vi "FIB realtime imaging PXIe-6124.vi"(0 "HW Config":T4={"FIB X coil"="FIB/ao0", "FIB Y coil"="FIB/ao1", "Beam blank"="FIB/port0/line0", "Ext Scan"="FIB/port0/line1", "Detector"="FIB/ai1", "Post #1up"="PXI1Slot2/ao0", "Post #1down"="PXI1Slot2/ao1", "Post #2up"="PXI1Slot2/ao2", "Post #2down"="PXI1Slot2/ao3"}, 1 "Options":T3 {"Scan mode" items=["Raster", "Serpentine"]; "Det" items=["Detector A", "Detector B"]}, 2 "Single scan":bool, 3 "Scan Para":T2={"X resolution"=512, "Z resolution"=512, "X center"=0.0, "Z center"=0.0, "X size (V)"=10.0, "Z size (V)"=10.0, "Frame line rampdown ratio"=-0.1, "Scan rate (Hz)"=2000000, "Oversampling"=2} {"Frame line rampdown ratio" min=-1.0 max=1.0 step=0.05 format="%.2g"; "Scan rate (Hz)" max=4000000 format="%#.6p"}, 4 "As subVi":bool, 5 "COM port":refnum<visa-resource-name>="COM1") -> (7 "Info & Status":T1={"Actual scan rate"=2000000.0, "X resolution with rampdown"=552, "Actual sample rate"=4000000.0, "Fetch backlog"=664878.0, "Total scan points"=276000, "Frame rate (/s)"=7} {"Fetch backlog" format="%#_6p"; "Actual sample rate" format="%#_6p"; "Actual scan rate" format="%#_4p"}, 10 "error out":errorcluster)   [LabVIEW 2018]
uses:
  <vilib>/DAQmx/write.llb/DAQmx Write (Analog 1D DBL NChan 1Samp).vi
  <vilib>/DAQmx/write.llb/DAQmx Write (Digital Wfm 1Chan NSamp).vi
  <vilib>/DAQmx/write.llb/DAQmx Write (Analog 2D DBL NChan NSamp).vi
  <vilib>/DAQmx/read.llb/DAQmx Read (Raw 1D I16).vi
  <vilib>/Analysis/2dsp.llb/Decimate (single shot, DBL).vi
  <vilib>/DAQmx/create/channels.llb/DAQmx Create Channel (AI-Voltage-Basic).vi
  <vilib>/DAQmx/create/channels.llb/DAQmx Create Channel (AO-Voltage-Basic).vi
  <vilib>/DAQmx/miscellaneous.llb/DAQmx Fill In Error Info.vi
  <vilib>/Waveform/DWDTOps.llb/DWDT Invert Digital.vi
  <vilib>/DAQmx/configure/timing.llb/DAQmx Timing (Sample Clock).vi
  <vilib>/DAQmx/create/channels.llb/DAQmx Create Channel (DO-Digital Output).vi
  <vilib>/DAQmx/create/channels.llb/DAQmx Create Channel (CO-Pulse Generation-Frequency).vi
  <vilib>/DAQmx/configure/trigger.llb/DAQmx Start Trigger (Digital Edge).vi
  <vilib>/Waveform/DWDTOps.llb/DWDT Uncompress Digital.vi
  <vilib>/Waveform/DWDTOps.llb/Digital Pattern Generator (Single Value).vi
  <vilib>/Analysis/NI_AALPro.lvlib
  <resource>/objmgr/daqmx.rc
panel:
  in  "Spot":bool
  in  "Api":refnum<k7>(container)
  out "Image shift":u32
  out "AI SampleClk.MaxRate":dbl
  in  "Sweep enabled":bool
  in  "Focus (V)":dbl min=-10.0 max=10.0 step=0.1 format="%.3g"
  in  "Sweep rate (Hz)":dbl=0.5 min=0.01 step=0.1 format="%0.2f"
  in  "Level #":u8
  in  "Sweep direction":bool
  in  "Angle (V)":dbl min=-10.0 max=10.0 step=0.1 format="%.3g"
  in  "Position (V)":dbl min=-10.0 max=10.0 step=0.1 format="%.3g"
  in  "Imbalance (V)":dbl min=-10.0 max=10.0 step=0.1 format="%.3f"
  out "Post #2down":tag
  out "Post #2up":tag
  out "Post #1down":tag
  out "Post #1up":tag
  out "Low blanked":bool
  in  "Machine Type":u8(ring) items=["Feiss", "NVision", "Jeiss"]
  out "Ext scan":tag
  out "Detector":tag="PXI1Slot7/ai0"
  out "FIB Y coil":tag="PXI1Slot7/ao1"
  out "FIB X coil":tag="PXI1Slot7/ao0"
  in  "Beam blanked":bool
  out "Beam blank":tag="PXI1Slot7/port0/line0"
  out "Oversampling":u16=2
  out "Scan rate (Hz)":u32=2000000
  out "Frame line rampdown ratio":dbl=0.1
  out "Y end":dbl=1.0
  out "X end":dbl=1.0
  out "Y start":dbl=-1.0
  out "X start":dbl=-1.0
  out "Y resolution":u32=500
  out "X resolution":u32=500
  out "Flip z":bool
  out "Flip x":bool
  out "Scan mode":u16
  out "Live image":i16[][](graph)
  in  "stop":bool=TRUE
  # "Flip"
  # "Scan coils"
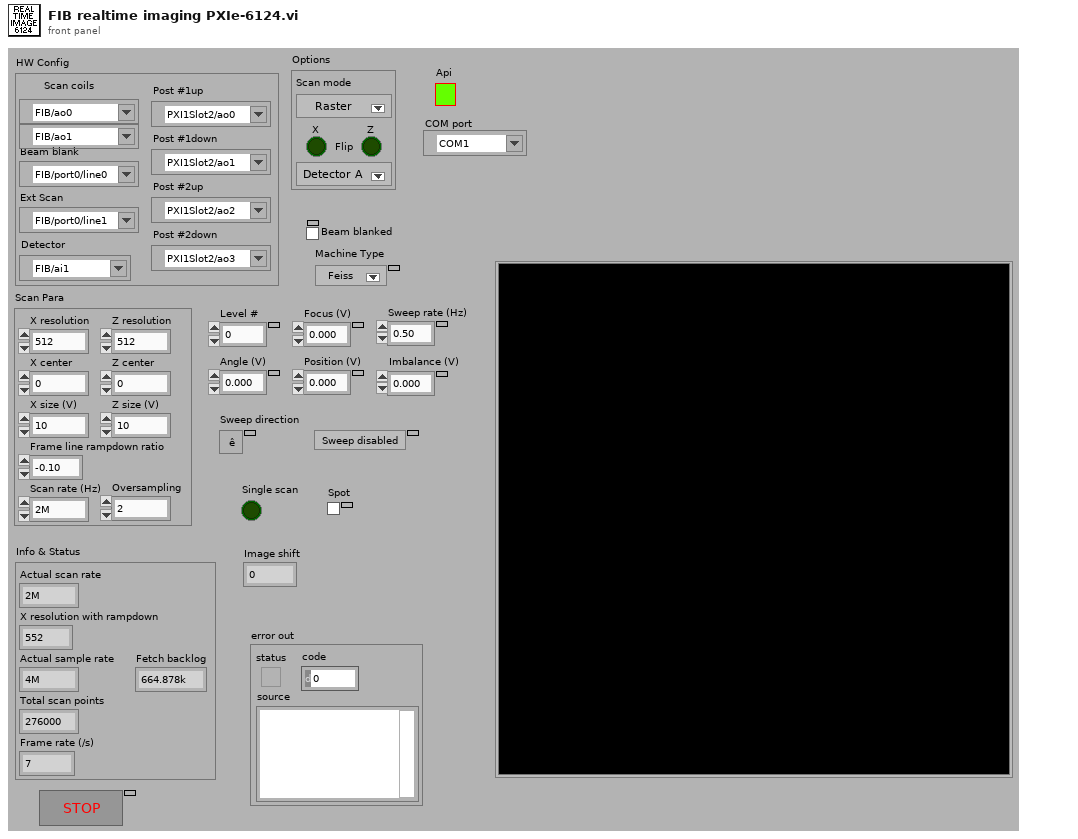
[diagram p1: front panel]
types:
  T1 = cluster{"Actual scan rate":dbl, "X resolution with rampdown":i32, "Actual sample rate":dbl, "Fetch backlog":dbl, "Total scan points":i32, "Frame rate (/s)":u32}
  T2 = cluster{"X resolution":u32, "Z resolution":u32, "X center":dbl, "Z center":dbl, "X size (V)":dbl, "Z size (V)":dbl, "Frame line rampdown ratio":dbl, "Scan rate (Hz)":u32, "Oversampling":u16}
  T3 = cluster{"Scan mode":u16, "Flip x":bool, "Flip z":bool, "Det":u16}
  T4 = cluster{"FIB X coil":tag, "FIB Y coil":tag, "Beam blank":tag, "Ext Scan":tag, "Detector":tag, "Post #1up":tag, "Post #1down":tag, "Post #2up":tag, "Post #2down":tag}
  T5 = enum16{"SEM", "FIB", "Milling", "SEM + FIB", "Mill + SEM", "SEM Drift Correction", "FIB Drift Correction", "No Beam", "External", "External + SEM"}
  T6 = enum16{"SEM", "FIB", "Mill", "SEM + FIB", "Mill + SEM", "Drift SEM", "Drift FIB", "None", "Ext", "Ext + SEM"}
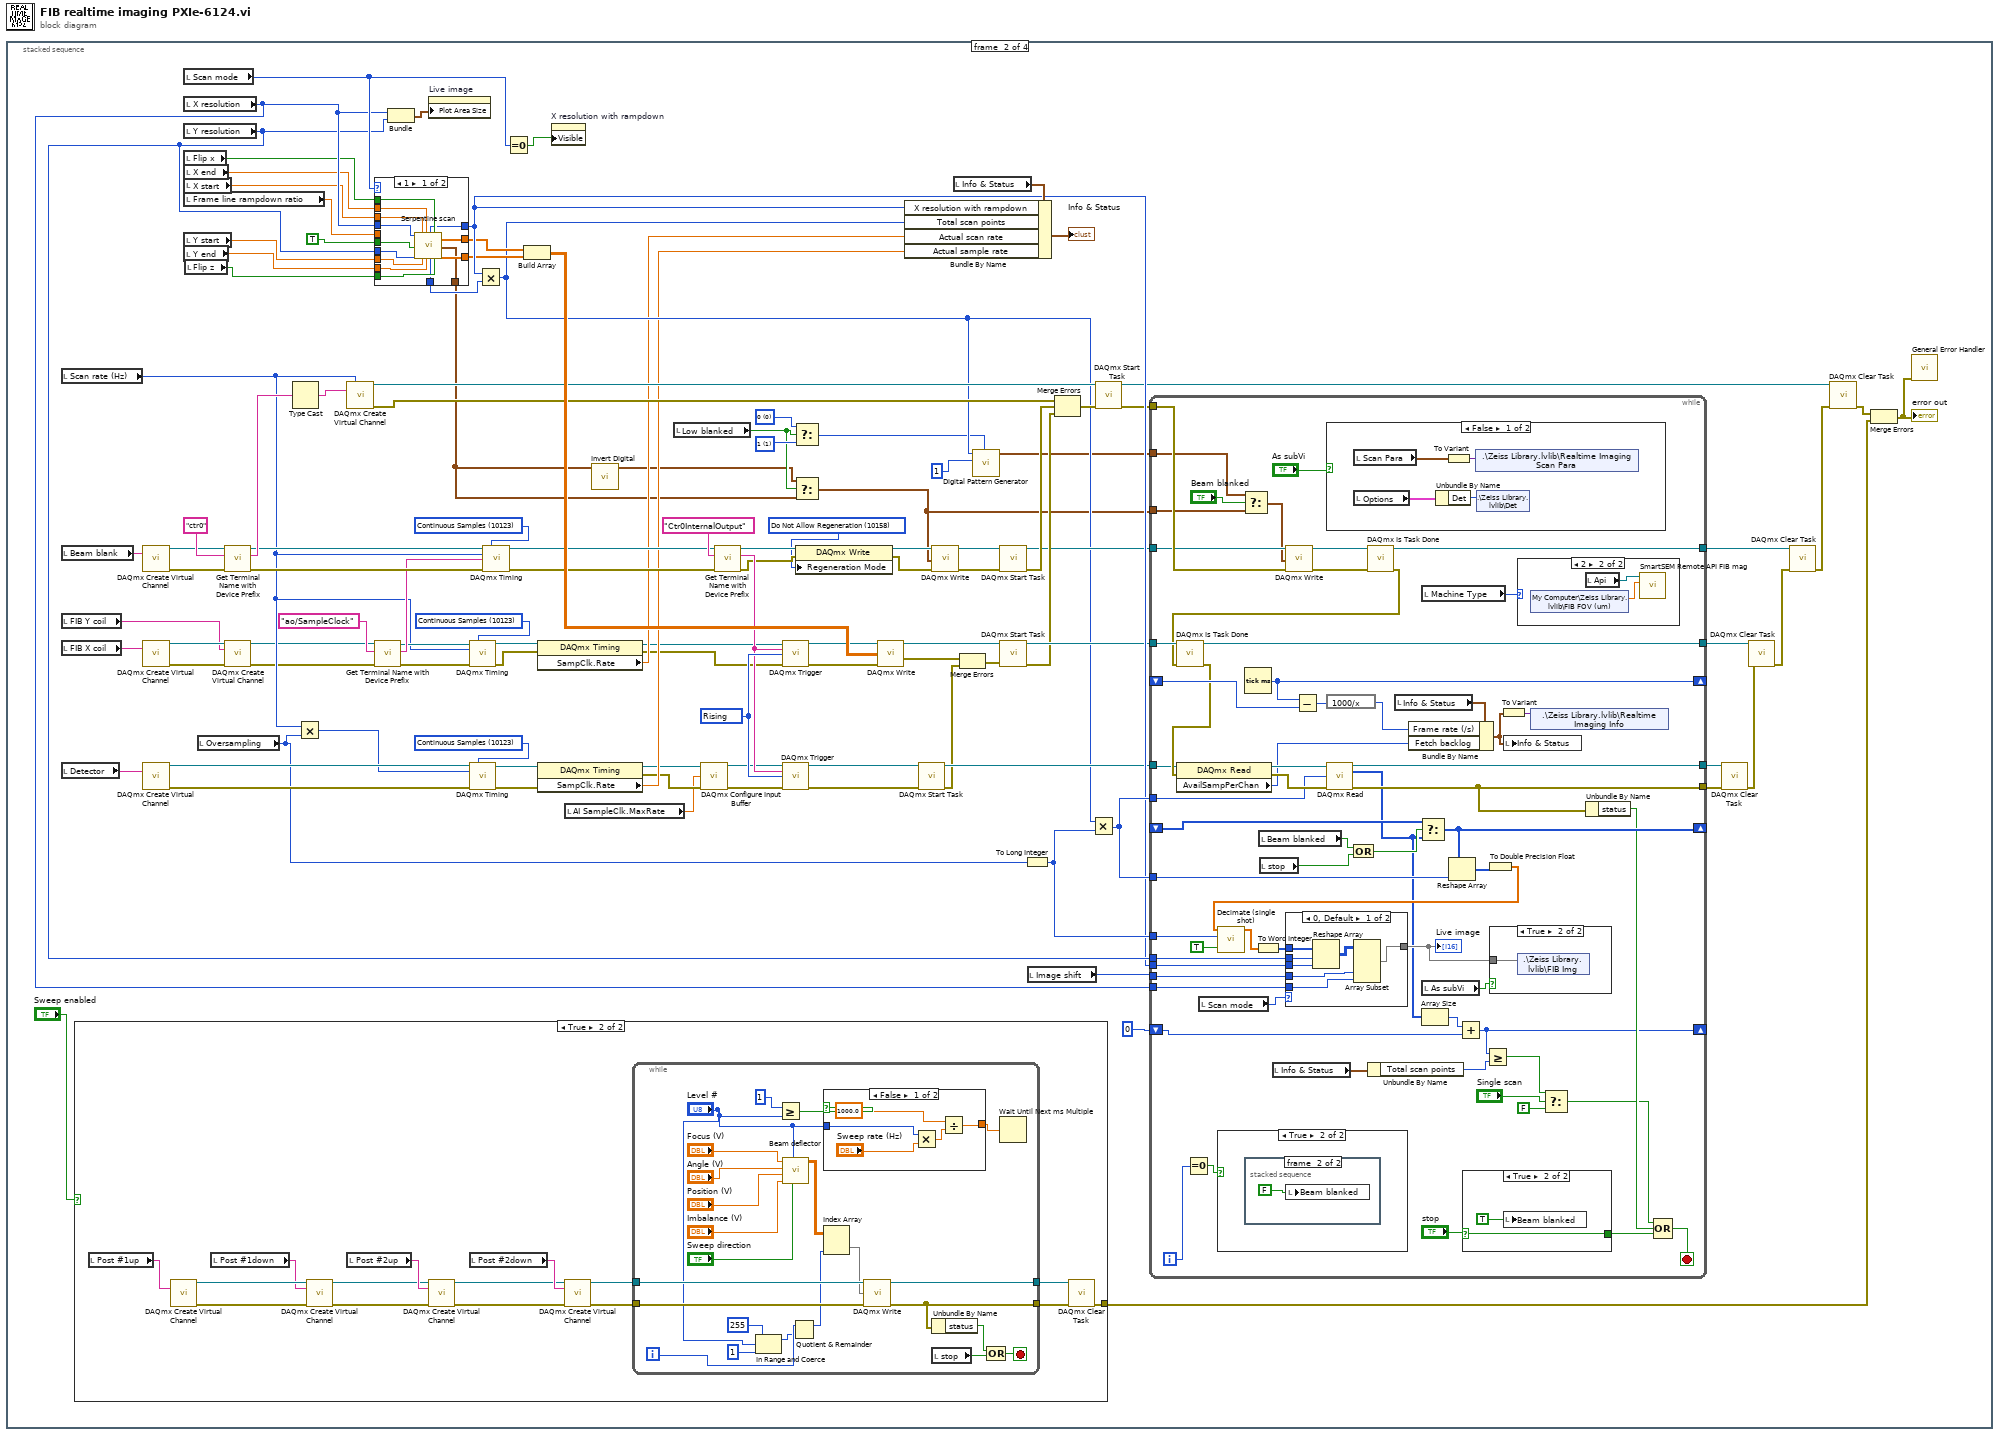
[diagram p0: block diagram]
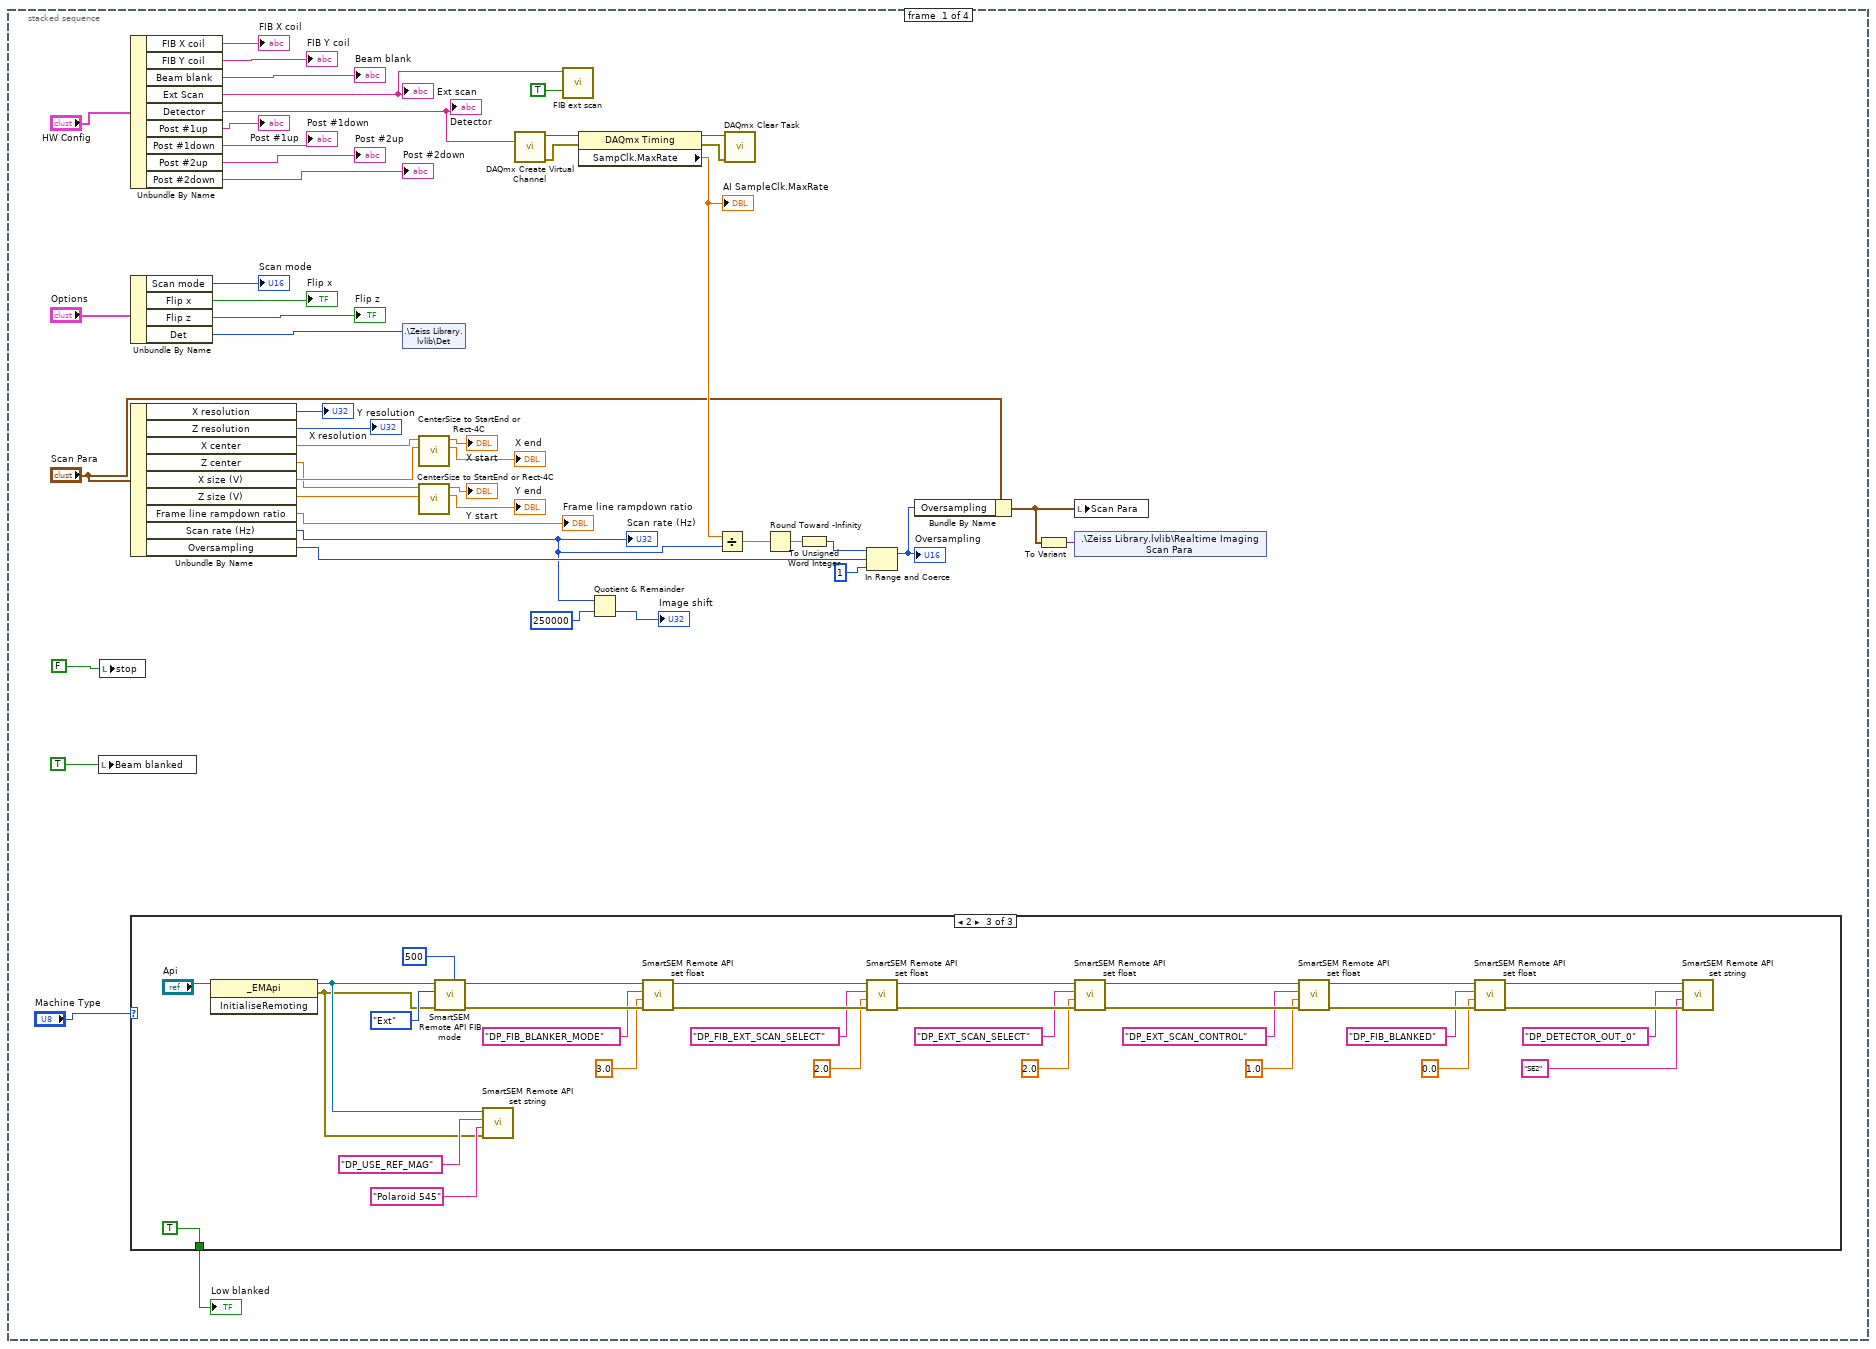
[diagram p2: hidden frame]
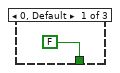
[diagram p3: hidden frame]
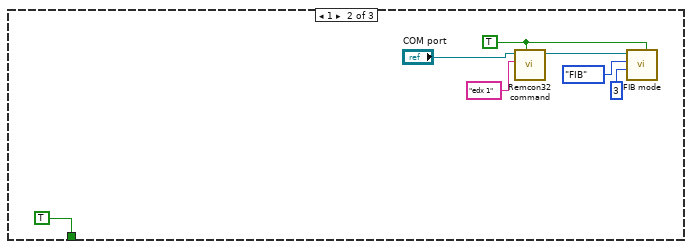
[diagram p4: hidden frame]
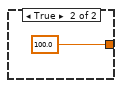
[diagram p6: hidden frame]
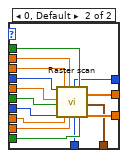
[diagram p7: hidden frame]
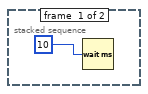
[diagram p11: hidden frame]
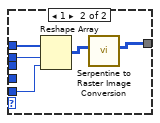
[diagram p14: hidden frame]
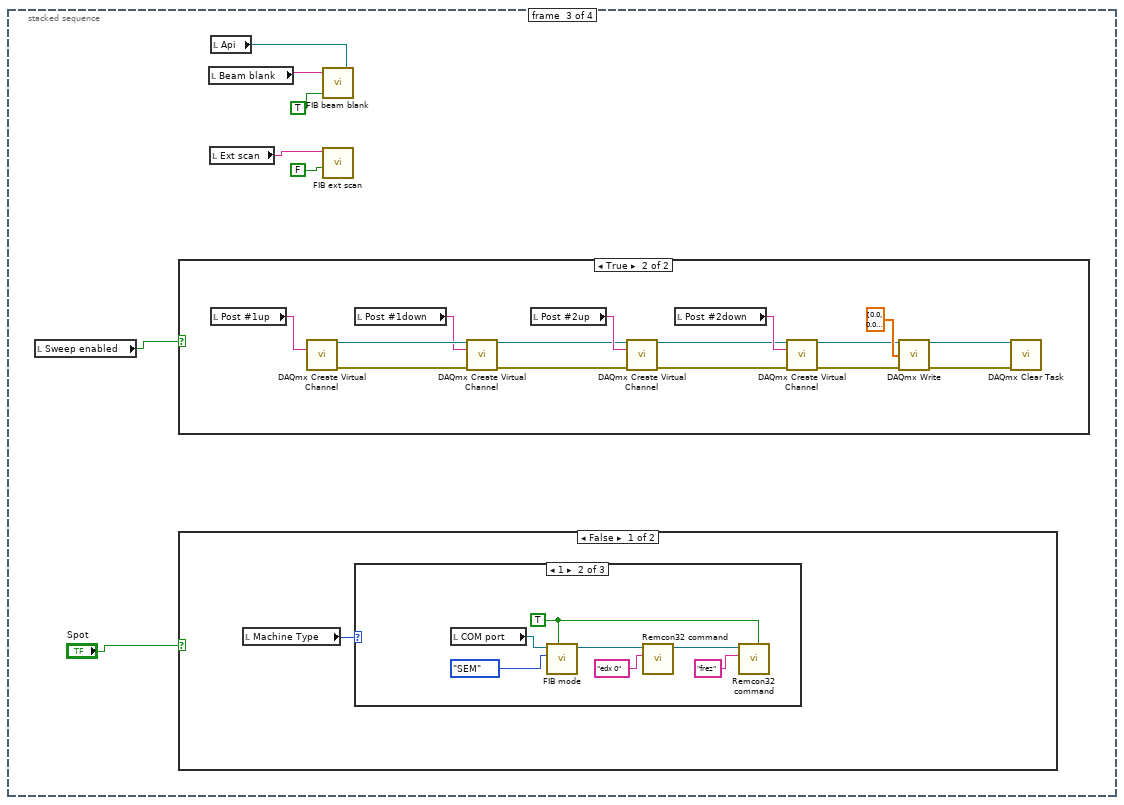
[diagram p15: hidden frame]
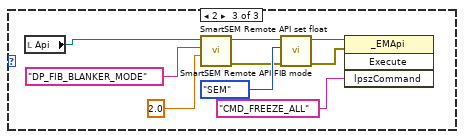
[diagram p17: hidden frame]
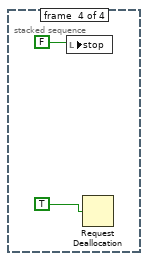
[diagram p20: hidden frame]
diagram:
  n1 = stacked-sequence {
    frame #0 {
      n2 = local write "Beam blanked"(TRUE ("Beam blanked")) -> ()
      n3 = local write "stop"(FALSE ("stop")) -> ()
      n4 = Unbundle By Name("HW Config") -> ("FIB X coil"=→"FIB X coil":tag, "FIB Y coil"=→"FIB Y coil":tag, "Beam blank"=→"Beam blank":tag, "Ext Scan"=w26:tag, "Detector"=w15:tag, "Post #1up"=→"Post #1up":tag, "Post #1down"=→"Post #1down":tag, "Post #2up"=→"Post #2up":tag, "Post #2down"=→"Post #2down":tag)
      "Detector" <- w15
      "Ext scan" <- w26
      n5 = Unbundle By Name("Options") -> ("Scan mode"=→"Scan mode":u16, "Flip x"=→"Flip x":bool, "Flip z"=→"Flip z":bool, "Det"=w40:u16)
      n6 = Unbundle By Name("Scan Para") -> ("X resolution"=→"X resolution":u32, "Z resolution"=→"Y resolution":u32, "X center"=w37:dbl, "Z center"=w33:dbl, "X size (V)"=w36:dbl, "Z size (V)"=w32:dbl, "Frame line rampdown ratio"=→"Frame line rampdown ratio":dbl, "Scan rate (Hz)"=w4:u32, "Oversampling"=w14:u16)
      "Scan rate (Hz)" <- w4
      n7 = case shown="2" "Machine Type" {
        tunnel: [FALSE ("Beam blanked") TRUE ("Beam blanked") TRUE ("Beam blanked")] -> w24
        frame 0, Default {
        }
        frame 1 {
          w53 = TRUE ("Close session")
          n8 = call "Remcon32 command.vi"("Initialization"=w53, "SEM command"="edx 1", "COM port in"="COM port") -> ("COM port out"=w52:refnum<visa-resource-name>)  [unwired: 5 in, 3 out]
          n9 = call "FIB mode.vi"("Close session"=w53, "Iterations"=u32 3, "FIB mode"=T5."FIB", "COM port in"=w52) -> ()  [unwired: 6 in, 2 out]
        }
        frame 2 {
          n10 = invoke class="_EMApi" method="InitialiseRemoting"(reference="Api") -> (reference out=w63:refnum<k7>, error out=w62:errorcluster)  [unwired: 2 in, 1 out]
          n11 = call "SmartSEM Remote API FIB mode.vi"("Wait (ms)"=u32 500, "error in"=w62, "FIB mode"=T6."Ext", "Api"=w63) -> ("error out"=w82:errorcluster, "Api out"=w83:refnum<k7>)  [unwired: 6 in]
          n12 = call "SmartSEM Remote API set string.vi"("error in"=w62, "vValue"="Polaroid 545" ("lpszParam"), "lpszParam"="DP_USE_REF_MAG", "Api"=w63) -> ()  [unwired: 6 in, 2 out]
          n13 = call "SmartSEM Remote API set float.vi"("error in"=w82, "vValue"=sgl 3.0, "lpszParam"="DP_FIB_BLANKER_MODE", "Api"=w83) -> ("error out"=w78:errorcluster, "Api out"=w79:refnum<k7>)  [unwired: 6 in]
          n14 = call "SmartSEM Remote API set float.vi"("error in"=w78, "vValue"=sgl 2.0, "lpszParam"="DP_FIB_EXT_SCAN_SELECT" ("lpszCommand"), "Api"=w79) -> ("error out"=w74:errorcluster, "Api out"=w75:refnum<k7>)  [unwired: 6 in]
          n15 = call "SmartSEM Remote API set float.vi"("vValue"=sgl 2.0, "lpszParam"="DP_EXT_SCAN_SELECT" ("lpszCommand")) -> ()  [unwired: 8 in, 2 out]
          n16 = call "SmartSEM Remote API set float.vi"("error in"=w74, "vValue"=sgl 1.0, "lpszParam"="DP_EXT_SCAN_CONTROL" ("lpszCommand"), "Api"=w75) -> ("error out"=w70:errorcluster, "Api out"=w71:refnum<k7>)  [unwired: 6 in]
          n17 = call "SmartSEM Remote API set float.vi"("error in"=w70, "vValue"=sgl 0.0, "lpszParam"="DP_FIB_BLANKED", "Api"=w71) -> ("error out"=w66:errorcluster, "Api out"=w67:refnum<k7>)  [unwired: 6 in]
          n18 = call "SmartSEM Remote API set string.vi"("error in"=w66, "vValue"="SE2" ("Det A Type"), "lpszParam"="DP_DETECTOR_OUT_0", "Api"=w67) -> ()  [unwired: 6 in, 2 out]
        }
      }
      "Low blanked" <- w24
      n19 = shared-variable ".\\Zeiss Library.lvlib\\Det"(w40) -> ()  [unwired: 1 in, 1 out]
      n20 = call "CenterSize to StartEnd or Rect-4C.vi"("Size"=w36, "Center"=w37) -> ("End"=→"X end":dbl, "Start"=→"X start":dbl)  [unwired: 3 in, 1 out]
      n21 = call "CenterSize to StartEnd or Rect-4C.vi"("Size"=w32, "Center"=w33) -> ("End"=→"Y end":dbl, "Start"=→"Y start":dbl)  [unwired: 3 in, 1 out]
      n22 = call-poly <vilib>:"DAQmx Create Virtual Channel.vi"("physical channels"=w15) -> ("task out"=w17:refnum<k21>, "error out"=w19:errorcluster)  [unwired: 8 in, 5 out]
      n23 = call "FIB ext scan.vi"("Ext on"=TRUE ("data"), "FIB Ext Scan"=w26) -> ()  [unwired: 9 in, 1 out]
      n24 = property class="DAQmx Timing"(reference=w17, error in=w19) -> (reference out=w16:refnum<k21>, error out=w18:errorcluster, "SampClk.MaxRate"=w12:dbl)
      "AI SampleClk.MaxRate" <- w12
      n25 = Quotient & Remainder(x=w4, y=u32 250000) -> (floor(x/y)=→"Image shift":u32)  [unwired: 1 out]
      n26 = Divide(x=w12, y=w4) -> (x/y=w11:dbl)
      n27 = call <vilib>:"DAQmx Clear Task.vi"("task in"=w16, "error in"=w18) -> ()  [unwired: 14 out]
      n28 = Round Toward -Infinity(1:w11) -> (0:w10:dbl)
      n29 = To Unsigned Word Integer(number=w10) -> (unsigned 16bit integer=w9:u16)
      n30 = In Range and Coerce(upper limit=w9, x=w14, lower limit=u16 1) -> (coerced(x)=w7:u16)  [unwired: 1 out]
      "Oversampling" <- w7
      n31 = Bundle By Name(cluster="Scan Para", "Oversampling"=w7) -> (w6:T2)
      n32 = To Variant(anything=w6) -> (Variant=w39:variant)
      n33 = local write "Scan Para"(w6) -> ()
      n34 = shared-variable ".\\Zeiss Library.lvlib\\Realtime Imaging Scan Para"(w39) -> ()  [unwired: 1 in, 1 out]
    }
    frame #1 {
      w105 = u8 1 items=["0", "1", "Z", "L", "H", "X", "T", "V"] ("value")
      w106 = u8 0 items=["0", "1", "Z", "L", "H", "X", "T", "V"] ("value")
      w117 = 10158 items=["Allow Regeneration"=10097, "Do Not Allow Regeneration"=10158] ("RegenMode")
      w142 = 10123 items=["Finite Samples"=10178, "Continuous Samples"=10123] ("sample mode")
      w130 = 10280 items=["Rising"=10280, "Falling"=10171] ("edge")
      w173 = 10123 items=["Finite Samples"=10178, "Continuous Samples"=10123, "Hardware Timed Single Point"=12522] ("sample mode")
      w177 = 10123 items=["Finite Samples"=10178, "Continuous Samples"=10123, "Hardware Timed Single Point"=12522] ("sample mode")
      n35 = local read "Scan rate (Hz)"() -> (w123:u32)
      n36 = local read "Beam blank"() -> (w111:tag)
      n37 = local read "FIB Y coil"() -> (w178:tag)
      n38 = local read "FIB X coil"() -> (w179:tag)
      n39 = local read "Detector"() -> (w180:tag)
      n40 = case shown="True" "Sweep enabled" {
        tunnel: [_ w216] -> w99
        frame False {
        }
        frame True {
          n41 = local read "Post #1up"() -> (w213:tag)
          n42 = call-poly <vilib>:"DAQmx Create Virtual Channel.vi"("physical channels"=w213) -> ("task out"=w215:refnum<k21>, "error out"=w214:errorcluster)  [unwired: 13 in]
          n43 = local read "Post #1down"() -> (w212:tag)
          n44 = call-poly <vilib>:"DAQmx Create Virtual Channel.vi"("task in"=w215, "physical channels"=w212, "error in"=w214) -> ("task out"=w203:refnum<k21>, "error out"=w202:errorcluster)  [unwired: 11 in]
          n45 = local read "Post #2up"() -> (w208:tag)
          n46 = call-poly <vilib>:"DAQmx Create Virtual Channel.vi"("task in"=w203, "physical channels"=w208, "error in"=w202) -> ("task out"=w206:refnum<k21>, "error out"=w207:errorcluster)  [unwired: 11 in]
          n47 = local read "Post #2down"() -> (w209:tag)
          n48 = call-poly <vilib>:"DAQmx Create Virtual Channel.vi"("task in"=w206, "physical channels"=w209, "error in"=w207) -> ("task out"=w205:refnum<k21>, "error out"=w204:errorcluster)  [unwired: 11 in]
          n49 = while {
            tunnel: [w235] -> w211
            tunnel: [w236] -> w210
            tunnel: w205 -> [w234]
            tunnel: w204 -> [w233]
            i -> [w231]
            stop <- w239 stop-if-true
            n50 = In Range and Coerce(upper limit=u8 255 ("lower limit"), x="Level #", lower limit=u8 1) -> (coerced(x)=w225:u8)  [unwired: 1 out]
            n51 = Greater Or Equal?(x=u8 1 ("y"), y="Level #") -> (x >= y?=w229:bool)
            n52 = call "Beam deflector.vi"("Sweep direction"="Sweep direction", "Level #"="Level #", "Imbalance (V)"="Imbalance (V)", "Position (V)"="Position (V)", "Angle (V)"="Angle (V)", "Focus (V)"="Focus (V)") -> ("All posts"=w218:dbl[][])  [unwired: 5 in]
            n53 = Quotient & Remainder(x=w231, y=w225) -> (x-y*floor(x/y)=w228:i32)  [unwired: 1 out]
            n54 = case shown="False" w229 {
              tunnel: "Level #" -> [w243 _]
              tunnel: [w240 100.0] -> w230
              frame False {
                n55 = Multiply(x=w243, y="Sweep rate (Hz)") -> (x*y=w242:dbl)
                n56 = Divide(x=1000.0, y=w242) -> (x/y=w240:dbl)
              }
              frame True {
              }
            }
            n57 = Index Array(array=w218, index (col)=w228) -> (element=w217:dbl[])  [unwired: 1 in]
            n58 = call-poly <vilib>:"DAQmx Write.vi"("task/channels in"=w234, "data"=w217, "error in"=w233) -> ("task out"=w236:refnum<k21>, "error out"=w235:errorcluster)  [unwired: 1 in, 10 out]
            n59 = Unbundle By Name(w235) -> ("status"=w237:bool)
            n60 = local read "stop"() -> (w238:bool)
            n61 = Compound Arithmetic op=OR(w237, w238) -> (w239:bool)
            n62 = Wait Until Next ms Multiple(millisecond multiple=w230) -> ()  [unwired: 1 out]
          }
          n63 = call <vilib>:"DAQmx Clear Task.vi"("task in"=w210, "error in"=w211) -> ("error out"=w216:errorcluster)  [unwired: 13 in]
        }
      }
      n64 = call-poly <vilib>:"DAQmx Create Virtual Channel.vi"("lines"=w111) -> ("task out"=w149:refnum<k21>, "error out"=w151:errorcluster)  [unwired: 6 in, 7 out]
      n65 = call-poly <vilib>:"DAQmx Create Virtual Channel.vi"("physical channels"=w179) -> ("task out"=w182:refnum<k21>, "error out"=w181:errorcluster)  [unwired: 8 in, 5 out]
      n66 = call-poly <vilib>:"DAQmx Create Virtual Channel.vi"("physical channels"=w180) -> ("task out"=w175:refnum<k21>, "error out"=w174:errorcluster)  [unwired: 8 in, 5 out]
      n67 = local read "Scan mode"() -> (w198:u16)
      n68 = local read "X resolution"() -> (w197:u32)
      n69 = local read "Y resolution"() -> (w196:u32)
      n70 = local read "Flip x"() -> (w188:bool)
      n71 = local read "X end"() -> (w185:dbl)
      n72 = local read "X start"() -> (w186:dbl)
      n73 = local read "Frame line rampdown ratio"() -> (w195:dbl)
      n74 = local read "Y start"() -> (w184:dbl)
      n75 = local read "Y end"() -> (w183:dbl)
      n76 = local read "Flip z"() -> (w187:bool)
      n77 = local read "Oversampling"() -> (w122:u16)
      n78 = call "Get Terminal Name with Device Prefix.vi"("error in"=w151, "Local Terminal Name"="ctr0", "task/channels in"=w149) -> ("error out"=w152:errorcluster, "Terminal Name with Device Prefix"=w154:tag, "task out"=w150:refnum<k21>)  [unwired: 6 in]
      n79 = call-poly <vilib>:"DAQmx Create Virtual Channel.vi"("task in"=w182, "physical channels"=w178, "error in"=w181) -> ("task out"=w90:refnum<k21>, "error out"=w89:errorcluster)  [unwired: 6 in, 5 out]
      n80 = Type Cast(x=w154) -> (*(type *) &x=w155:string)  [unwired: 1 in]
      n81 = Multiply(x=w123, y=w122) -> (x*y=w124:u32)
      n82 = call-poly <vilib>:"DAQmx Create Virtual Channel.vi"("frequency"=w123, "counter"=w155) -> ("task out"=w145:refnum<k21>, "error out"=w147:errorcluster)  [unwired: 7 in, 5 out]
      n83 = case shown="1" w198 {
        tunnel: w195 -> [_ w271]
        tunnel: w188 -> [w254 w274]
        tunnel: w196 -> [w257 w269]
        tunnel: w197 -> [w259 w272]
        tunnel: w187 -> [w251 w273]
        tunnel: [w250 w268] -> w191
        tunnel: [w249 w267] -> w190
        tunnel: TRUE ("Flip x") -> [w258 w270]
        tunnel: w186 -> [w256 w266]
        tunnel: w185 -> [w255 w265]
        tunnel: w184 -> [w253 w264]
        tunnel: w183 -> [w252 w263]
        tunnel: [w248 w262] -> w168
        tunnel: [w247 w261] -> w167
        tunnel: [w246 w260] -> w91
        frame 1 {
          n84 = call "Serpentine scan.vi"("X resolution"=w259, "Scan pattern?"=w258, "Y resolution"=w257, "X start"=w256, "Y start"=w253, "X end"=w255, "Y end"=w252, "Flip x"=w254, "Flip y"=w251) -> ("X resolution with rampdown"=w250:i32, "Y resolution"=w249:i32, "X scan pattern"=w248:dbl[], "Blanking pattern"=w246:digitalwaveform, "Y scan pattern"=w247:dbl[])  [unwired: 3 in, 3 out]
        }
        frame 0, Default {
          n85 = call "Raster scan.vi"("X resolution"=w272, "Frame line rampdown ratio"=w271, "Scan pattern?"=w270, "Y resolution"=w269, "X start"=w266, "Y start"=w264, "X end"=w265, "Y end"=w263, "Flip x"=w274, "Flip y"=w273) -> ("X resolution with rampdown"=w268:i32, "Y resolution"=w267:i32, "X scan pattern"=w262:dbl[], "Blanking pattern"=w260:digitalwaveform, "Y scan pattern"=w261:dbl[])  [unwired: 2 in, 3 out]
        }
      }
      n86 = call "Get Terminal Name with Device Prefix.vi"("error in"=w89, "Local Terminal Name"="ao/SampleClock", "task/channels in"=w90) -> ("error out"=w125:errorcluster, "Terminal Name with Device Prefix"=w138:tag, "task out"=w126:refnum<k21>)  [unwired: 6 in]
      n87 = Bundle("X resolution"=w197, "Y resolution"=w196) -> (w200:cluster{"X resolution":u32, "Y resolution":u32})  [unwired: 1 in]
      n88 = property on="Live image" class="IntGraph (strict)"("Plot Area Size"=w200) -> ()  [unwired: 2 in, 2 out]
      n89 = call-poly <vilib>:"DAQmx Timing.vi"("task/channels in"=w126, "sample mode"=w177, "rate"=w123, "error in"=w125) -> ("task out"=w128:refnum<k21>, "error out"=w127:errorcluster)  [unwired: 3 in, 7 out]
      n90 = call-poly <vilib>:"DAQmx Timing.vi"("task/channels in"=w175, "sample mode"=w173, "rate"=w124, "error in"=w174) -> ("task out"=w172:refnum<k21>, "error out"=w171:errorcluster)  [unwired: 3 in, 7 out]
      n91 = Multiply(x=w191, y=w190) -> (x*y=w115:i32)
      n92 = call-poly <vilib>:"DAQmx Timing.vi"("task/channels in"=w150, "sample mode"=w142, "rate"=w123, "source"=w138, "error in"=w152) -> ("task out"=w141:refnum<k21>, "error out"=w140:errorcluster)  [unwired: 2 in, 7 out]
      n93 = Equal To 0?(x=w198) -> (x = 0?=w192:bool)
      n94 = Build Array(w168, w167) -> (w166:dbl[][])
      n95 = property class="DAQmx Timing"(reference=w128, error in=w127) -> (reference out=w108:refnum<k21>, error out=w107:errorcluster, "SampClk.Rate"=w110:dbl)
      n96 = property class="DAQmx Timing"(reference=w172, error in=w171) -> (reference out=w97:refnum<k21>, error out=w94:errorcluster, "SampClk.Rate"=w109:dbl)
      n97 = property on="X resolution with rampdown" class="DigNum (strict)"("Visible"=w192) -> ()  [unwired: 2 in, 2 out]
      n98 = local read "AI SampleClk.MaxRate"() -> (w93:dbl)
      n99 = call-poly <vilib>:"Invert Digital.vi"("digital waveform"=w91) -> ("inverted waveform"=w92:digitalwaveform)  [unwired: 9 in, 1 out]
      n100 = local read "Low blanked"() -> (w102:bool)
      n101 = call <vilib>:"DAQmx Configure Input Buffer.vi"("task/channels in"=w97, "buffer size (in samples per channel)"=w93, "error in"=w94) -> ("task out"=w96:refnum<k21>, "error out"=w95:errorcluster)  [unwired: 11 in]
      n102 = call "Get Terminal Name with Device Prefix.vi"("error in"=w140, "Local Terminal Name"="Ctr0InternalOutput" ("terminal"), "task/channels in"=w141) -> ("error out"=w119:errorcluster, "Terminal Name with Device Prefix"=w129:tag, "task out"=w121:refnum<k21>)  [unwired: 1 in, 5 out]
      n103 = call-poly <vilib>:"DAQmx Trigger.vi"("task/channels in"=w108, "source"=w129, "edge"=w130, "error in"=w107) -> ("task out"=w131:refnum<k21>, "error out"=w132:errorcluster)  [unwired: 10 out]
      n104 = call-poly <vilib>:"DAQmx Trigger.vi"("task/channels in"=w96, "source"=w129, "edge"=w130, "error in"=w95) -> ("task out"=w170:refnum<k21>, "error out"=w169:errorcluster)  [unwired: 10 out]
      n105 = Select(t=w106, s=w102, f=w105) -> (s? t:f=w104:u8)
      n106 = Select(t=w92, s=w102, f=w91) -> (s? t:f=w103:digitalwaveform)
      n107 = property class="DAQmx Write"(reference=w121, error in=w119, "Regeneration Mode"=w117) -> (reference out=w120:refnum<k21>, error out=w118:errorcluster)
      n108 = call-poly <vilib>:"DAQmx Write.vi"("task/channels in"=w131, "data"=w166, "error in"=w132) -> ("task out"=w165:refnum<k21>, "error out"=w163:errorcluster)  [unwired: 1 in, 10 out]
      n109 = call <vilib>:"DAQmx Start Task.vi"("task/channels in"=w170, "error in"=w169) -> ("task out"=w162:refnum<k21>, "error out"=w161:errorcluster)  [unwired: 12 out]
      n110 = call-poly <vilib>:"DAQmx Write.vi"("task/channels in"=w120, "data"=w103, "error in"=w118) -> ("task out"=w144:refnum<k21>, "error out"=w139:errorcluster)  [unwired: 2 in, 9 out]
      n111 = local read "Info & Status"() -> (w194:T1)
      n112 = Bundle By Name(cluster=w194, "X resolution with rampdown"=w191, "Total scan points"=w115, "Actual scan rate"=w110, "Actual sample rate"=w109) -> (→"Info & Status":T1)
      n113 = Merge Errors(w163, w161) -> (w164:errorcluster)
      n114 = call-poly <vilib>:"Digital Pattern Generator.vi"("value"=w104, "number of signals"=u32 1, "number of samples"=w115) -> ("digital waveform"=w114:digitalwaveform)  [unwired: 2 in, 6 out]
      n115 = call <vilib>:"DAQmx Start Task.vi"("task/channels in"=w144, "error in"=w139) -> ("task out"=w135:refnum<k21>, "error out"=w146:errorcluster)  [unwired: 12 out]
      n116 = call <vilib>:"DAQmx Start Task.vi"("task/channels in"=w165, "error in"=w164) -> ("task out"=w160:refnum<k21>, "error out"=w137:errorcluster)  [unwired: 12 out]
      n117 = To Long Integer(number=w122) -> (32bit integer=w201:i32)
      n118 = local read "Image shift"() -> (w87:u32)
      n119 = Merge Errors(w147, w146, w137) -> (w148:errorcluster)
      n120 = Multiply(x=w115, y=w201) -> (x*y=w199:i32)
      n121 = call <vilib>:"DAQmx Start Task.vi"("task/channels in"=w145, "error in"=w148) -> ("task out"=w134:refnum<k21>, "error out"=w136:errorcluster)  [unwired: 12 out]
      n122 = while {
        shift-right: [w332] -> _
        shift-left: _ -> [w331]
        tunnel: w201 -> [w330]
        tunnel: w196 -> [w329]
        tunnel: w191 -> [w328]
        tunnel: w197 -> [w327]
        tunnel: w199 -> [w298]
        tunnel: w199 -> [w326]
        shift-right: [w309] -> _
        shift-left: _ -> [w317]
        tunnel: w162 -> [w300]
        tunnel: w160 -> [w308]
        tunnel: [w307] -> w158
        tunnel: [w306] -> w159
        tunnel: [w305] -> w157
        tunnel: w136 -> [w293]
        tunnel: w135 -> [w292]
        tunnel: [w296] -> w133
        tunnel: w103 -> [w290]
        tunnel: w114 -> [w289]
        shift-right: [w283] -> _
        shift-left: 0 -> [w285]
        tunnel: w87 -> [w276]
        i -> [w310]
        stop <- w338 stop-if-true
        n123 = Equal To 0?(x=w310) -> (x = 0?=w311:bool)
        n124 = local read "Scan mode"() -> (w325:u16)
        n125 = case shown="True" w311 {
          frame False {
          }
          frame True {
            n126 = stacked-sequence {
              frame #0 {
                n127 = Wait (ms)(milliseconds to wait=u32 10) -> ()  [unwired: 1 out]
              }
              frame #1 {
                n128 = local write "Beam blanked"(FALSE ("Beam blanked")) -> ()
              }
            }
          }
        }
        n129 = Select(t=w289, s="Beam blanked", f=w290) -> (s? t:f=w277:digitalwaveform)
        n130 = Tick Count (ms)() -> (millisecond timer value=w332:u32)
        n131 = local read "Beam blanked"() -> (w314:bool)
        n132 = local read "stop"() -> (w312:bool)
        n133 = local read "Info & Status"() -> (w284:T1)
        n134 = call-poly <vilib>:"DAQmx Write.vi"("task/channels in"=w292, "data"=w277, "error in"=w293) -> ("task out"=w291:refnum<k21>, "error out"=w294:errorcluster)  [unwired: 2 in, 9 out]
        n135 = Subtract(x=w332, y=w331) -> (x-y=w319:u32)
        n136 = case shown="False" "As subVi" {
          frame False {
            n137 = local read "Scan Para"() -> (w341:T2)
            n138 = local read "Options"() -> (w344:T3)
            n139 = Unbundle By Name(w344) -> ("Det"=w343:u16)
            n140 = To Variant(anything=w341) -> (Variant=w342:variant)
            n141 = shared-variable ".\\Zeiss Library.lvlib\\Realtime Imaging Scan Para"(w342) -> ()  [unwired: 1 in, 1 out]
            n142 = shared-variable ".\\Zeiss Library.lvlib\\Det"(w343) -> ()  [unwired: 1 in, 1 out]
          }
          frame True {
          }
        }
        n143 = expression code="1000/x"(w319) -> (w322:u32)
        n144 = Compound Arithmetic op=OR(w314, w312) -> (w313:bool)
        n145 = call <vilib>:"DAQmx Is Task Done.vi"("task/channels in"=w291, "error in"=w294) -> ("task out"=w296:refnum<k21>, "error out"=w297:errorcluster)  [unwired: 2 in, 10 out]
        n146 = call <vilib>:"DAQmx Is Task Done.vi"("task/channels in"=w308, "error in"=w297) -> ("task out"=w305:refnum<k21>, "error out"=w303:errorcluster)  [unwired: 2 in, 10 out]
        n147 = property class="DAQmx Read"(reference=w300, error in=w303) -> (reference out=w301:refnum<k21>, error out=w302:errorcluster, "AvailSampPerChan"=w299:u32)
        n148 = call-poly <vilib>:"DAQmx Read.vi"("task/channels in"=w301, "number of samples per channel"=w298, "error in"=w302) -> ("task out"=w306:refnum<k21>, "data"=w287:i16[], "error out"=w307:errorcluster)  [unwired: 10 out]
        n149 = Unbundle By Name(w284) -> ("Total scan points"=w282:i32)
        n150 = local read "Info & Status"() -> (w323:T1)
        n151 = Bundle By Name(cluster=w323, "Frame rate (/s)"=w322, "Fetch backlog"=w299) -> (w320:T1)
        n152 = Select(t=w317, s=w313, f=w287) -> (s? t:f=w309:i16[])
        n153 = local read "Machine Type"() -> (w275:u8)
        n154 = local read "As subVi"() -> (w318:bool)
        n155 = Array Size(array=w287) -> (size(s)=w286:i32)
        n156 = Reshape Array(w309, w326) -> (w334:i16[])
        n157 = Add(x=w286, y=w285) -> (x+y=w283:i32)
        n158 = case shown="True" "stop" {
          selector: "stop" -> [w347 w349]
          tunnel: [w347 w349] -> w315
          frame False {
          }
          frame True {
            n159 = local write "Beam blanked"(TRUE ("Beam blanked")) -> ()
          }
        }
        n160 = Greater Or Equal?(x=w283, y=w282) -> (x >= y?=w280:bool)
        n161 = To Double Precision Float(number=w334) -> (double precision float=w333:dbl[])
        n162 = call-poly <vilib>:"Decimate (single shot).vi"("averaging"=TRUE, "decimating factor"=w330, "X"=w333) -> ("Decimated Array"=w336:dbl[])  [unwired: 8 out]
        n163 = To Word Integer(number=w336) -> (16bit integer=w335:i16[])
        n164 = case shown="0, Default" w325 {
          tunnel: w335 -> [w357 w362]
          tunnel: w329 -> [w355 w361]
          tunnel: w328 -> [w354 _]
          tunnel: w327 -> [w353 w360]
          tunnel: [w352 w358] -> w324
          tunnel: w276 -> [w351 _]
          frame 0, Default {
            n165 = Reshape Array(w357, w355, w354) -> (w356:i16[][])
            n166 = Array Subset(array=w356, index (col)=w351, length (col)=w353) -> (w352:i16[][])  [unwired: 2 in]
          }
          frame 1 {
            n167 = Reshape Array(w362, w361, w360) -> (w359:i16[][])
            n168 = call "Serpentine to Raster Image Conversion.vi"("Input"=w359) -> ("Output"=w358:i16[][])  [unwired: 10 in]
          }
        }
        "Live image" <- w324
        n169 = case shown="True" w318 {
          tunnel: w324 -> [_ w350]
          frame False {
          }
          frame True {
            n170 = shared-variable ".\\Zeiss Library.lvlib\\FIB Img"(w350) -> ()  [unwired: 1 in, 1 out]
          }
        }
        n171 = To Variant(anything=w320) -> (Variant=w321:variant)
        n172 = local write "Info & Status"(w320) -> ()
        n173 = case shown="2" w275 {
          frame 0, Default {
          }
          frame 2 {
            n174 = shared-variable "My Computer\\Zeiss Library.lvlib\\FIB FOV (um)"() -> (w339:sgl)  [unwired: 1 in, 1 out]
            n175 = local read "Api"() -> (w340:refnum<k7>)
            n176 = call "SmartSEM Remote API FIB mag.vi"("FIB FOV (um)"=w339, "Api"=w340) -> ()  [unwired: 8 in, 2 out]
          }
        }
        n177 = shared-variable ".\\Zeiss Library.lvlib\\Realtime Imaging Info"(w321) -> ()  [unwired: 1 in, 1 out]
        n178 = Select(t=w280, s="Single scan", f=FALSE) -> (s? t:f=w278:bool)
        n179 = Unbundle By Name(w307) -> ("status"=w304:bool)
        n180 = Compound Arithmetic op=OR(w278, w304, w315) -> (w338:bool)
      }
      n181 = call <vilib>:"DAQmx Clear Task.vi"("task in"=w159, "error in"=w158) -> ("error out"=w156:errorcluster)  [unwired: 13 out]
      n182 = call <vilib>:"DAQmx Clear Task.vi"("task in"=w157, "error in"=w156) -> ("error out"=w113:errorcluster)  [unwired: 13 out]
      n183 = call <vilib>:"DAQmx Clear Task.vi"("task in"=w133, "error in"=w113) -> ("error out"=w112:errorcluster)  [unwired: 13 out]
      n184 = call <vilib>:"DAQmx Clear Task.vi"("task in"=w134, "error in"=w112) -> ("error out"=w100:errorcluster)  [unwired: 13 out]
      n185 = Merge Errors(w100, w99) -> (w101:errorcluster)
      "error out" <- w101
      n186 = call <vilib>:"General Error Handler.vi"("error in (no error)"=w101) -> ()  [unwired: 10 in, 5 out]
    }
    frame #2 {
      n187 = local read "Sweep enabled"() -> (w365:bool)
      n188 = case shown="True" w365 {
        frame False {
        }
        frame True {
          n189 = local read "Post #1up"() -> (w396:tag)
          n190 = call-poly <vilib>:"DAQmx Create Virtual Channel.vi"("physical channels"=w396) -> ("task out"=w398:refnum<k21>, "error out"=w397:errorcluster)  [unwired: 13 in]
          n191 = local read "Post #1down"() -> (w395:tag)
          n192 = call-poly <vilib>:"DAQmx Create Virtual Channel.vi"("task in"=w398, "physical channels"=w395, "error in"=w397) -> ("task out"=w388:refnum<k21>, "error out"=w387:errorcluster)  [unwired: 11 in]
          n193 = local read "Post #2up"() -> (w393:tag)
          n194 = call-poly <vilib>:"DAQmx Create Virtual Channel.vi"("task in"=w388, "physical channels"=w393, "error in"=w387) -> ("task out"=w391:refnum<k21>, "error out"=w392:errorcluster)  [unwired: 11 in]
          n195 = local read "Post #2down"() -> (w394:tag)
          n196 = call-poly <vilib>:"DAQmx Create Virtual Channel.vi"("task in"=w391, "physical channels"=w394, "error in"=w392) -> ("task out"=w390:refnum<k21>, "error out"=w389:errorcluster)  [unwired: 11 in]
          n197 = call-poly <vilib>:"DAQmx Write.vi"("task/channels in"=w390, "data"=dbl[] [0.0, 0.0, 0.0, 0.0], "error in"=w389) -> ("task out"=w399:refnum<k21>, "error out"=w400:errorcluster)  [unwired: 1 in, 10 out]
          n198 = call <vilib>:"DAQmx Clear Task.vi"("task in"=w399, "error in"=w400) -> ()  [unwired: 13 in, 1 out]
        }
      }
      n199 = case shown="False" "Spot" {
        frame False {
          n200 = local read "Machine Type"() -> (w370:u8)
          n201 = case shown="1" w370 {
            frame 0, Default {
            }
            frame 1 {
              w377 = TRUE ("Initialization")
              n202 = local read "COM port"() -> (w371:refnum<visa-resource-name>)
              n203 = call "FIB mode.vi"("Initialization"=w377, "FIB mode"=T5."SEM", "COM port in"=w371) -> ("COM port out"=w372:refnum<visa-resource-name>)  [unwired: 7 in, 1 out]
              n204 = call "Remcon32 command.vi"("SEM command"="edx 0", "COM port in"=w372) -> ("COM port out"=w373:refnum<visa-resource-name>)  [unwired: 6 in, 3 out]
              n205 = call "Remcon32 command.vi"("Close session"=w377, "SEM command"="frez", "COM port in"=w373) -> ()  [unwired: 5 in, 4 out]
            }
            frame 2 {
              n206 = local read "Api"() -> (w382:refnum<k7>)
              n207 = call "SmartSEM Remote API set float.vi"("vValue"=sgl 2.0, "lpszParam"="DP_FIB_BLANKER_MODE" ("lpszCommand"), "Api"=w382) -> ("error out"=w378:errorcluster, "Api out"=w379:refnum<k7>)  [unwired: 7 in]
              n208 = call "SmartSEM Remote API FIB mode.vi"("error in"=w378, "FIB mode"=T6."SEM", "Api"=w379) -> ("error out"=w383:errorcluster, "Api out"=w384:refnum<k7>)  [unwired: 7 in]
              n209 = invoke class="_EMApi" method="Execute"(reference=w384, error in=w383, "lpszCommand"="CMD_FREEZE_ALL") -> ()  [unwired: 1 in, 4 out]
            }
          }
        }
        frame True {
        }
      }
      n210 = local read "Beam blank"() -> (w368:tag)
      n211 = local read "Ext scan"() -> (w367:tag)
      n212 = local read "Api"() -> (w363:refnum<k7>)
      n213 = call "FIB beam blank.vi"("Api"=w363, "Beam blanked"=TRUE, "lines"=w368) -> ()  [unwired: 2 in, 1 out]
      n214 = call "FIB ext scan.vi"("Ext on"=FALSE ("data"), "FIB Ext Scan"=w367) -> ()  [unwired: 9 in, 1 out]
    }
    frame #3 {
      n215 = local write "stop"(FALSE ("stop")) -> ()
      n216 = Request Deallocation(TRUE ("flag")) -> ()
    }
  }
